vi "Write VI Refnum.vi"(8 "Error In":errorcluster, 10 "VI Refnum":refnum<vi>, 11 "NumericOperation in":refnum<class "NumericOperation.lvclass">) -> (0 "Error Out":errorcluster, 3 "NumericOperation out":refnum<class "NumericOperation.lvclass">)   [LabVIEW 2021, in "Calculator.lvlib" / "NumericOperation.lvclass"]
uses:
  NumericOperation.lvclass
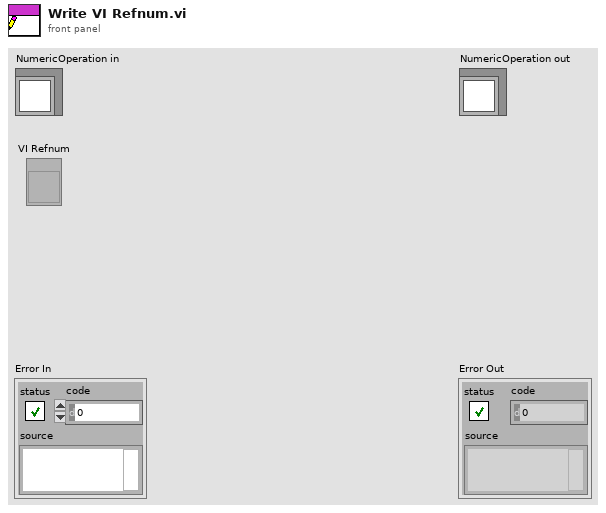
[diagram p1: front panel]
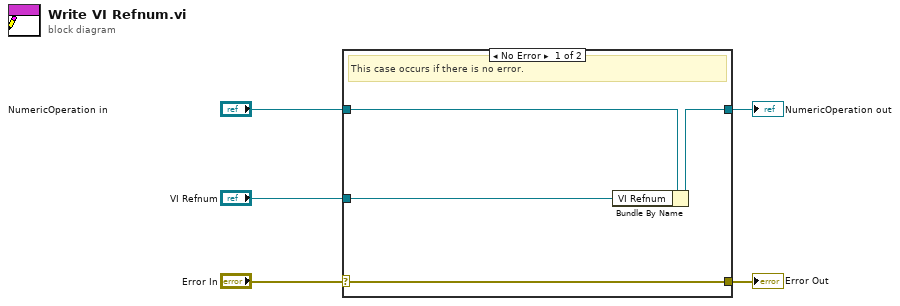
[diagram p0: block diagram]
diagram:
  n1 = case shown="No Error" "Error In" {
    selector: "Error In" -> [w9 w10]
    tunnel: [w9 w10] -> w4
    tunnel: [w7 w11] -> w2
    tunnel: "NumericOperation in" -> [w8 w11]
    tunnel: "VI Refnum" -> [w6 _]
    frame No Error {
      # "This case occurs if there is no error."
      n2 = Bundle By Name(cluster=w8, "VI Refnum"=w6) -> (w7:refnum<class "NumericOperation.lvclass">)
    }
    frame Error {
      # "This  case occurs if there is any error."
    }
  }
  "Error Out" <- w4
  "NumericOperation out" <- w2
